vi "rx_ed.vi"(11 "Wavefrom":cluster{"t0":dbl, "dt":dbl, cdb[]}) -> (0 "first pulse":i32, 1 "debug":dbl[](array[numeric]), 2 "length":i32[](array[numeric]), 3 "start index":i32[](array[numeric]))   [LabVIEW 2014]
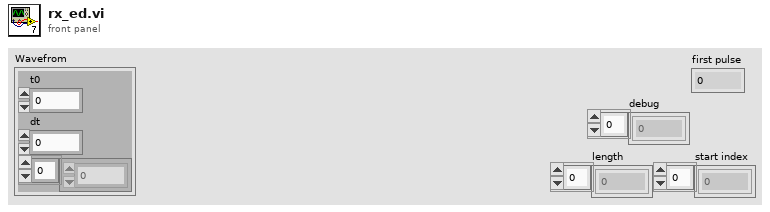
[diagram p1: front panel]
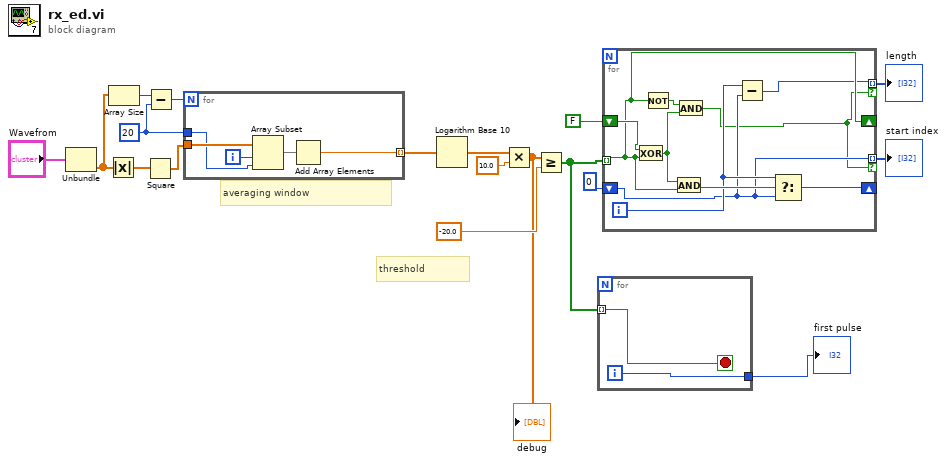
[diagram p0: block diagram]
diagram:
  w14 = 20 ("y")
  # "averaging window"
  # "threshold"
  n1 = Unbundle("Wavefrom") -> (w9:cdb[])  [unwired: 2 out]
  n2 = Absolute Value(x=w9) -> (abs(x)=w16:dbl[])
  n3 = Array Size(array=w9) -> (size(s)=w18:i32)
  n4 = Square(x=w16) -> (x^2=w15:dbl[])
  n5 = Subtract(x=w18, y=w14) -> (x-y=w17:i32)
  n6 = for {
    N: w17 -> [_]
    tunnel: w15 -> [w23]
    tunnel: w14 -> [w21]
    tunnel: [w19] -> w13 mode=indexing
    i -> [w22]
    n7 = Array Subset(array=w23, index=w22, length=w21) -> (w20:dbl[])
    n8 = Add Array Elements(numeric array=w20) -> (sum=w19:dbl)
  }
  n9 = Logarithm Base 10(1:w13) -> (0:w12:dbl[])
  n10 = Multiply(x=w12, y=10.0) -> (x*y=w3:dbl[])
  "debug" <- w3
  n11 = Greater Or Equal?(x=w3, y=-20.0) -> (x >= y?=w2:bool[])
  n12 = for {
    tunnel: w2 -> [w25] mode=indexing
    tunnel: [w24] -> w1
    i -> [w24]
    stop <- w25 stop-if-true
  }
  "first pulse" <- w1
  n13 = for {
    tunnel: w2 -> [w29] mode=indexing
    shift-right: [w29] -> _
    shift-left: FALSE -> [w35]
    shift-right: [w31] -> _
    shift-left: 0 -> [w28]
    tunnel: [w28] -> w4 mode=indexing if=w26
    tunnel: [w27] -> w5 mode=indexing if=w26
    i -> [w30]
    n14 = Exclusive Or(1:w29, 2:w35) -> (0:w33:bool)
    n15 = Not(x=w29) -> (.not. x?=w34:bool)
    n16 = And(x=w33, y=w29) -> (x .and. y?=w32:bool)
    n17 = And(x=w34, y=w33) -> (x .and. y?=w26:bool)
    n18 = Subtract(x=w30, y=w28) -> (x-y=w27:i32)
    n19 = Select(t=w30, s=w32, f=w28) -> (s? t:f=w31:i32)
  }
  "length" <- w5
  "start index" <- w4
